vi "Speaker.vi"() -> ()   [LabVIEW 2019]
doc: "Speaker"
uses:
  <vilib>/sound2/lvsound2.llb/Sound Data Format.ctl
  <vilib>/sound2/lvsound2.llb/Sampling Mode.ctl
  <vilib>/sound2/lvsound2.llb/Sound Output Write (DBL Single).vi
  <vilib>/Analysis/NI_AALBase.lvlib
panel:
  in  "stop":bool
  in  "Frequncy":dbl
  out "error out 2":errorcluster
  in  "sound format":T1={"sample rate (S/s)"=22050.0, "number of channels"=2, "bits per sample"=16}
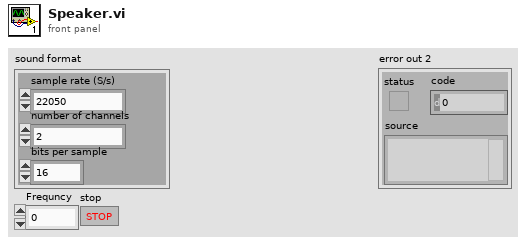
[diagram p1: front panel]
types:
  T1 = typedef "Sound Data Format.ctl" = cluster{"sample rate (S/s)":dbl, "number of channels":i32, "bits per sample":i32}
  T2 = typedef "Sampling Mode.ctl" = i32
  T3 = typedef "Sound Output Task ID.ctl" = u32
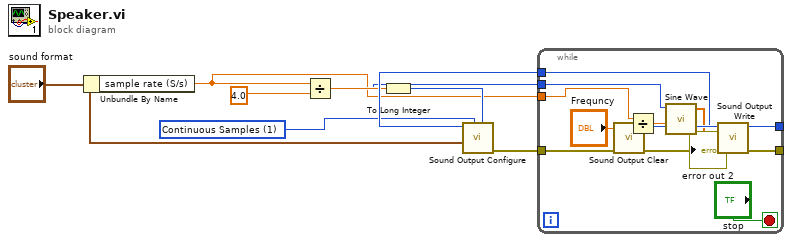
[diagram p0: block diagram]
diagram:
  w5 = T2 1 items=["Finite Samples", "Continuous Samples"] ("sample mode")
  n1 = Unbundle By Name("sound format") -> ("sample rate (S/s)"=w1:dbl)
  n2 = Divide(x=w1, y=4.0) -> (x/y=w3:dbl)
  n3 = To Long Integer(number=w3) -> (32bit integer=w2:i32)
  n4 = call <vilib>:"Sound Output Configure.vi"("number of samples/ch"=w2, "sample mode"=w5, "sound format"="sound format") -> ("error out"=w10:errorcluster, "task ID"=w7:T3)  [unwired: 7 in]
  n5 = while {
    tunnel: w10 -> [w21]
    tunnel: [w20] -> w9
    tunnel: w7 -> [w19]
    tunnel: [w18] -> w6
    tunnel: w2 -> [w17]
    tunnel: w1 -> [w12]
    stop <- "stop" stop-if-true
    n6 = Divide(x=w12, y="Frequncy") -> (x/y=w16:dbl)
    n7 = call <vilib>:"Sine Wave.vi"("samples"=w17, "frequency"=w16) -> ("sine wave"=w15:dbl[])  [unwired: 3 in, 2 out]
    n8 = call-poly <vilib>:"Sound Output Write.vi"("error in (no error)"=w21, "data"=w15, "task ID"=w19) -> ("error out"=w20:errorcluster, "task ID out"=w18:T3)  [unwired: 7 in]
  }
  n9 = call <vilib>:"Sound Output Clear.vi"("error in (no error)"=w9, "task ID"=w6) -> ("error out"=→"error out 2":errorcluster)  [unwired: 9 in]
